vi "get refnums.vi"(8 "error in (no error)":errorcluster, 11 "Elevator Concrete in":refnum<class "Elevator Concrete.lvclass">) -> (0 "error out":errorcluster, 1 "Motor refnums":T1, 3 "Elevator Concrete out":refnum<class "Elevator Concrete.lvclass">)   [LabVIEW 2018, in "Elevator.lvlib" / "Elevator Concrete.lvclass"]
uses:
  Elevator Concrete.lvclass
  Elevator Concrete.lvclass/Elevator Concrete.ctl
  Elevator.lvclass
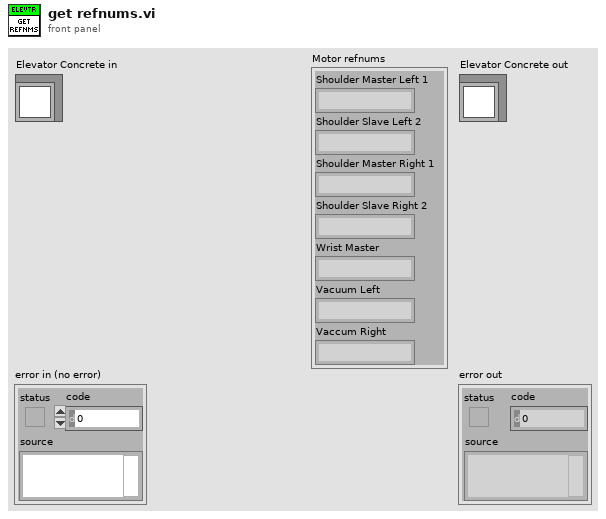
[diagram p1: front panel]
types:
  T1 = cluster{"Shoulder Master Left 1":string, "Shoulder Slave Left 2":string, "Shoulder Master Right 1":string, "Shoulder Slave Right 2 ":string, "Wrist Master ":string, "Vacuum Left":string, "Vaccum Right":string}
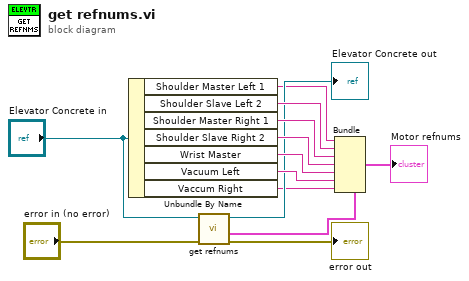
[diagram p0: block diagram]
diagram:
  n1 = Unbundle By Name("Elevator Concrete in") -> ("Shoulder Master Left 1"=w2:string, "Shoulder Slave Left 2"=w12:string, "Shoulder Master Right 1"=w11:string, "Shoulder Slave Right 2"=w10:string, "Wrist Master"=w9:string, "Vacuum Left"=w8:string, "Vaccum Right"=w1:string)
  n2 = call-parent "get refnums.vi"("error in (no error)"="error in (no error)", "Elevator in"="Elevator Concrete in") -> ("error out"=→"error out":errorcluster, "motor refnums"=w4:T1, "Elevator out"=→"Elevator Concrete out":refnum<class "Elevator Concrete.lvclass">)  [unwired: 7 in]
  n3 = Bundle(cluster=w4, "Shoulder Master Left 1"=w2, "Shoulder Slave Left 2"=w12, "Shoulder Master Right 1"=w11, "Shoulder Slave Right 2"=w10, "Wrist Master"=w9, "Vacuum Left"=w8, "Vaccum Right"=w1) -> (→"Motor refnums":T1)
